vi "Data Matrix Grading AIM DPM 2006.vi"() -> ()   [LabVIEW 2014]
doc: "This example illustrates AIM DPM-2006 Data Matrix grading functionality.\n\nVision Development Module support three Data Matrix grading standards: ISO/IEC 16022-2000, ISO/IEC 15415-2004, and AIM DPM-2006. Run this VI. You can adjust the delay to slow down execution."
uses:
  <vilib>/vision/Instrument.llb/Data Matrix Search Options.ctl
  <vilib>/vision/Instrument.llb/Demodulation Mode.ctl
  <vilib>/vision/Instrument.llb/Cell Sample Size.ctl
  <vilib>/vision/Instrument.llb/Cell Filter Mode.ctl
  <vilib>/vision/Instrument.llb/Data Matrix Description Options.ctl
  <vilib>/vision/Instrument.llb/ECC Type.ctl
  <vilib>/vision/Instrument.llb/Data Matrix Polarity.ctl
  <vilib>/vision/Instrument.llb/Cell Fill Percentage.ctl
  <vilib>/vision/Instrument.llb/Data Matrix Mirror.ctl
  <vilib>/vision/Instrument.llb/Data Matrix Size Options.ctl
  <vilib>/vision/Instrument.llb/Data Matrix Advanced Options.ctl
  <vilib>/vision/Instrument.llb/Prepare For Grading.ctl
  <vilib>/vision/NI_Vision_Development_Module.lvlib
panel:
  out "AIM DPM Grading Report":T1
  out "Barcode Type":string
  in  "Stop":bool
  in  "Delay (s.)":dbl(slide)=0.4897959183673469 scale=0.0..2.0
  out "Read Time (ms)":dbl format="%.2f"
  out "Data":string
  out "Image":T2(plugin-control)
  # "Overview: Demonstrate the use of the Data Matrix AIM DPM-2006 grading feature.\nRequirements: Vision Development Module\nInstructions: Run the VI."
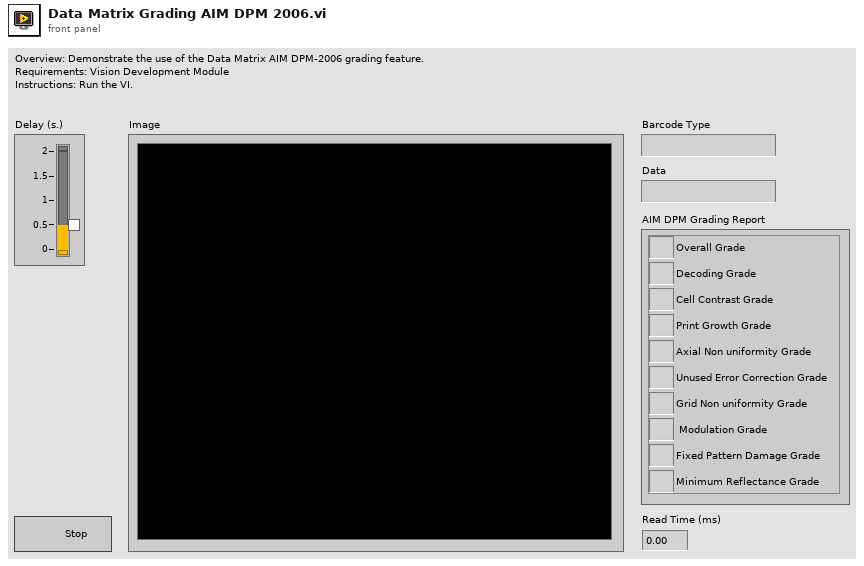
[diagram p1: front panel]
types:
  T1 = cluster{"Overall Grade":string, "Decoding Grade":string, "Cell Contrast Grade":string, "Print Growth Grade":string, "Axial Non uniformity Grade":string, "Unused Error Correction Grade":string, "Grid Non uniformity Grade":string, " Modulation Grade":string, "Fixed Pattern Damage Grade":string, "Minimum Reflectance Grade":string}
  T2 = typedef "IMAQ Image.ctl" = refnum<image>
  T3 = typedef "Data Matrix Advanced Options.ctl" = cluster{"Option":enum32{"Line Detection", "HighLight Filter", "Aggressive", "FNC1", "Refine Bounding Box"}, " Value":dbl}
  T4 = typedef "Data Matrix Size Options.ctl" = cluster{"Data Matrix Size":cluster{"Minimum Size":u32, "Maximum Size":u32}, "Quiet Zone Width":u32}
  T5 = typedef "Data Matrix Description Options.ctl" = cluster{"Aspect Ratio":sgl, "Rows":u32, "Columns":u32, "Rectangle":bool, "ECC":T6, "Barcode Polarity":T7, "Cell Fill Percentage":T8, "Minimum Border Integrity %":sgl, "Mirror Mode":T9}
  T6 = typedef "ECC Type.ctl" = i32
  T7 = typedef "Data Matrix Polarity.ctl" = i32
  T8 = typedef "Cell Fill Percentage.ctl" = i32
  T9 = typedef "Data Matrix Mirror.ctl" = i32
  T10 = typedef "Data Matrix Search Options.ctl" = cluster{"Rotation Mode":enum32{"Unlimited", "0 Degrees", "90 Degrees", "180 Degrees", "270 Degrees"}, "Skip Location?":bool, "Edge Threshold":u32, "Demodulation Mode":T11, "Cell Sample Size":T12, "Cell Filter Mode":T13, "Skew Degrees Allowed":u32, "Maximum Iterations":u32, "Initial Search Vector Width":u32}
  T11 = typedef "Demodulation Mode.ctl" = i32
  T12 = typedef "Cell Sample Size.ctl" = i32
  T13 = typedef "Cell Filter Mode.ctl" = i32
  T14 = typedef "Prepare For Grading.ctl" = i32
  T15 = typedef "Data Matrix Report.ctl" = cluster{"Found?":bool, "Binary?":bool, "Data":string, "Bounding Box":cluster{"x":sgl, "y":sgl}[], "Errors Corrected":u32, "Erasures Corrected":u32, "Aspect Ratio":sgl, "Rows":u32, "Columns":u32, "ECC":T6, "Barcode Polarity":T7, "Cell Fill Percentage":T8, "Border Integrity":sgl, "Mirrored?":bool, "Minimum Edge Strength":u32, "Demodulation Mode":T11, "Cell Sample Size":T12, "Cell Filter Mode":T13, "Iterations":u32}
  T16 = typedef "Data Matrix AIM Grade.ctl" = string
  T17 = cluster{"Overall Grade":T16, "Decoding Grade":T16, "Cell Contrast Grade":T16, "Print Growth Grade":T16, "Axial Nonuniformity Grade":T16, "Unused Error Correction Grade":T16, "Grid Nonuniformity Grade":T16, " Modulation Grade":T16, "Fixed Pattern Damage Grade":T16, "Minimum Reflectance Grade":T16}
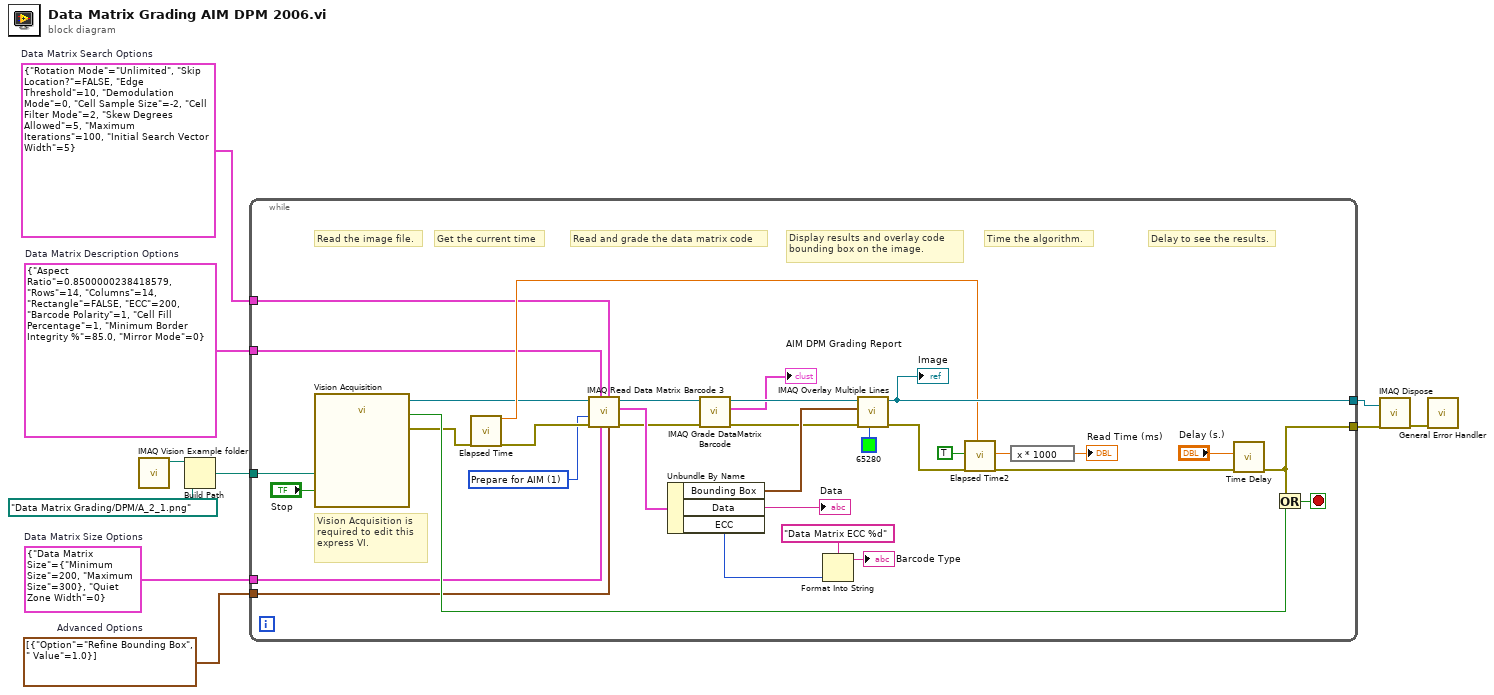
[diagram p0: block diagram]
diagram:
  w1 = T3[] [{"Option"=enum."Refine Bounding Box", " Value"=1.0}]  # Advanced Options
  w2 = T4 {"Data Matrix Size"={"Minimum Size"=200, "Maximum Size"=300}, "Quiet Zone Width"=0}  # Data Matrix Size Options
  w4 = T5 {"Aspect Ratio"=0.85, "Rows"=14, "Columns"=14, "Rectangle"=FALSE, "ECC"=200, "Barcode Polarity"=1, "Cell Fill Percentage"=1, "Minimum Border Integrity %"=85.0, "Mirror Mode"=0}  # Data Matrix Description Options
  w3 = T10 {"Rotation Mode"=enum."Unlimited", "Skip Location?"=FALSE, "Edge Threshold"=10, "Demodulation Mode"=0, "Cell Sample Size"=-2, "Cell Filter Mode"=2, "Skew Degrees Allowed"=5, "Maximum Iterations"=100, "Initial Search Vector Width"=5}  # Data Matrix Search Options
  n1 = call "IMAQ Vision Example folder.vi"() -> ("Example Image Path"=w7:path)  [unwired: 11 in]
  n2 = Build Path(base path=w7, name or relative path=path "Data Matrix Grading/DPM/A_2_1.png" ("appended path")) -> (appended path=w5:path)
  n3 = while {
    tunnel: [w43] -> w10
    tunnel: [w42] -> w9
    tunnel: w5 -> [w38]
    tunnel: w4 -> [w19]
    tunnel: w3 -> [w18]
    tunnel: w2 -> [w17]
    tunnel: w1 -> [w16]
    stop <- w41 stop-if-true
    w11 = T14 1 items=["Do Not Prepare", "Prepare for AIM"] ("Prepare for Grading?")
    # "Vision Acquisition is required to edit this express VI."
    # "Delay to see the results."
    # "Time the algorithm."
    # "Read and grade the data matrix code"
    # "Get the current time"
    # "Read the image file."
    # "Display results and overlay code bounding box on the image."
    n4 = call "Vision Acquisition"("Image Path"=w38, "Stop (F)"="Stop") -> ("Image Out"=w25:T2, "Stopped"=w39:bool, "error out"=w23:errorcluster)  [unwired: 23 in]
    n5 = call "Elapsed Time"("error in (no error)"=w23) -> ("Present (s)"=w36:dbl, "error out"=w22:errorcluster)  [unwired: 11 in, 6 out]
    n6 = call "IMAQ Read Data Matrix Barcode 3"("Advanced Options"=w16, "Data Matrix Search Options"=w18, "Data Matrix Size Options"=w17, "Data Matrix Description Options"=w19, "error in (no error)"=w22, "Prepare for Grading?"=w11, "Image"=w25) -> ("error out"=w27:errorcluster, "Data Matrix Report"=w30:T15, "Image (duplicate)"=w29:T2)  [unwired: 1 in, 1 out]
    n7 = Unbundle By Name(w30) -> ("Bounding Box"=w31:cluster{"x":sgl, "y":sgl}[], "Data"=→"Data":string, "ECC"=w14:T6)
    n8 = call-poly "IMAQ Grade DataMatrix Barcode"("error in (no error)"=w27, "Image"=w29) -> ("error out"=w26:errorcluster, "AIM DPM Grading Report"=→"AIM DPM Grading Report":T17, "Image (duplicate)"=w28:T2)  [unwired: 1 in, 6 out]
    n9 = Format Into String(format string="Data Matrix ECC %d", w14) -> (resulting string=→"Barcode Type":string)  [unwired: 2 in, 1 out]
    n10 = call "IMAQ Overlay Multiple Lines"("Color"=u32 65280, "error in (no error)"=w26, "Line End Points"=w31, "Image"=w28) -> ("error out"=w34:errorcluster, "Image Out"=w43:T2)  [unwired: 2 in, 4 out]
    "Image" <- w43
    n11 = call "Elapsed Time2"("Reset"=TRUE, "error in (no error)"=w34, "Set Start Time (s)"=w36) -> ("Elapsed Time (s)"=w21:dbl, "error out"=w37:errorcluster)  [unwired: 9 in, 6 out]
    n12 = expression code="x * 1000"(w21) -> (→"Read Time (ms)":dbl)
    n13 = call "Time Delay"("error in (no error)"=w37, "Delay Time (s)"="Delay (s.)") -> ("error out"=w42:errorcluster)  [unwired: 9 in]
    n14 = Or(x=w42, y=w39) -> (x .or. y?=w41:bool)
  }
  n15 = call "IMAQ Dispose"("Image"=w10, "error in (no error)"=w9) -> ("error out"=w8:errorcluster)  [unwired: 1 in, 3 out]
  n16 = call <vilib>:"General Error Handler.vi"("error in (no error)"=w8) -> ()  [unwired: 10 in, 5 out]
